vi "Movement.vi"(0 "Rotational Speed":dbl, 1 "Sideways Speed":dbl, 2 "Forward Speed":dbl) -> ()   [LabVIEW 2013]
doc: "Controls movement of the robot. Just put in forward, sideways, and/or rotational speed and it will do everything else. This DOES use the gyro correction, so if you just put in a forward or sideways speed, it will use the gyro to keep you straight.\n\nSigns are as follows:\n- Back\n+ Forward\n\n- Slide Left\n+ Slide Right\n\n- Spin Left\n+ Sping Right"
uses:
  <vilib>/Rock Robotics/WPI/RobotDrive/WPI_RobotDriveMecanumDrive_Cartesian.vi
  <vilib>/Rock Robotics/WPI/RobotDrive/WPI_RobotDriveGetSetRefNum.vi
panel:
  # "-Back\n+Forward"
  # "-Left\n+Right"
  # "-Left\n+Right"
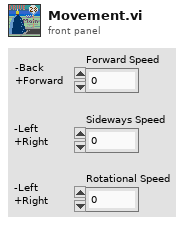
[diagram p1: front panel]
types:
  T1 = typedef "WPI_RobotDriveDevRef.ctl" = cluster{"DevStatus":errorcluster, "Motors[]":T2[], "Square Inputs":bool, "Max Output":dbl, "Isochronous":bool}
  T2 = typedef "WPI_MotorControlDeviceRef.ctl" = cluster{"DeviceStatus":errorcluster, "Type":enum16{"PWM", "CAN"}, "PWM":cluster{"Digital Module":T3, "PWM Channel":T4, "DeadBand":T5}, "CAN":cluster{"Device Number":u8, "Control Mode":T6, "Semaphore":T7, "Max Vout":dbl}, "Invert":bool, "TransformRef":T8, "InvTransformRef":T8}
  T3 = typedef "FPGA_TypedefDigitalModule.ctl" = enum16{"Digital Module 1", "Digital Module 2"}
  T4 = typedef "FPGA_DIOPWMChannel.ctl" = enum8{"PWM 1", "PWM 2", "PWM 3", "PWM 4", "PWM 5", "PWM 6", "PWM 7", "PWM 8", "PWM 9", "PWM 10", "Invalid"}
  T5 = typedef "WPI_PWMDeadband.ctl" = cluster{"Name":string, "maxPositivePwm":i32, "minPositivePwm":i32, "centerPwm":i32, "maxNegativePwm":i32, "minNegativePwm":i32, "angularRange":u16}
  T6 = typedef "WPI_CANJaguar_ControlMode.ctl" = enum8{"Percent VBus", "Current", "Speed", "Position", "Voltage"}
  T7 = typedef "Semaphore RefNum" = refnum<k1>
  T8 = typedef "WPI_PWMTransform_ConPane.ctl" = refnum<vi>
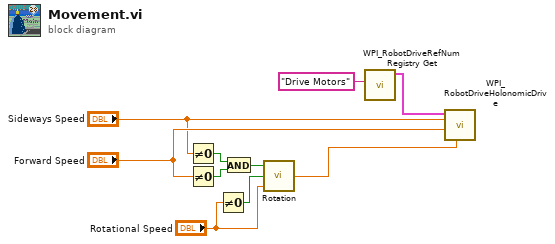
[diagram p0: block diagram]
diagram:
  n1 = Not Equal To 0?(x="Sideways Speed") -> (x != 0?=w6:bool)
  n2 = Not Equal To 0?(x="Forward Speed") -> (x != 0?=w5:bool)
  n3 = Not Equal To 0?(x="Rotational Speed") -> (x != 0?=w4:bool)
  n4 = And(x=w6, y=w5) -> (x .and. y?=w7:bool)
  n5 = call "Rotation.vi"("Uncorrected Speed"="Rotational Speed", "Rotating Manually"=w4, "Moving Laterally"=w7) -> ("Output Speed"=w8:dbl)
  n6 = call <vilib>:"WPI_RobotDriveRefNum Registry Get.vi"("refnum name"="Drive Motors") -> ("RobotDriveDevRef"=w10:T1)  [unwired: 1 in, 9 out]
  n7 = call-poly <vilib>:"WPI_RobotDriveHolonomicDrive.vi"("Rotation"=w8, "Y"="Forward Speed", "X"="Sideways Speed", "RobotDriveDevRef"=w10) -> ()  [unwired: 5 in, 3 out]
